vi "sample1.vi"() -> ()   [LabVIEW 2015]
uses:
  <vilib>/rvi/Emulation/niFpgaGetClockAttributes.vi
  <vilib>/rvi/Emulation/niFpgaSctlEmulationGetInTimedLoop.vi
  <vilib>/rvi/Emulation/niFpgaEmulationReportErrorSimple.vi
  <vilib>/rvi/eio/common/nirviEmuTemplateMethod_errors.vi
  <vilib>/rvi/Emulation/niFpgaCriticalErrorInLSC.vi
  <vilib>/rvi/Emulation/niFpgaProcessEmulError.vi
  <vilib>/eio/EIONode/EIONode.xnode
panel:
  in  "B Duty":u32 caption="Count(mSec)"
  in  "OR Duty":u32 caption="Count(mSec)"
  in  "OL Duty":u32 caption="Count(mSec)"
  in  "R duty":u32 caption="Count(mSec)"
  in  "Lights Period":u32
  in  "W duty":u32 caption="Count(mSec)"
  in  "Wiper Duty":u32 caption="Count(mSec)"
  in  "DoorB Duty":u32 caption="Count(mSec)"
  in  "Servo Period":u32
  in  "DoorA Duty":u32 caption="Count(mSec)"
  in  "Pulse Width":u32 caption="Count(mSec)"
  in  "Steering":i16
  in  "Stepper ON":bool
  in  "Period":u32=1
  in  "DIRECTION":bool
  in  "GAS":sgl
  in  "Count(mSec)":u32=1
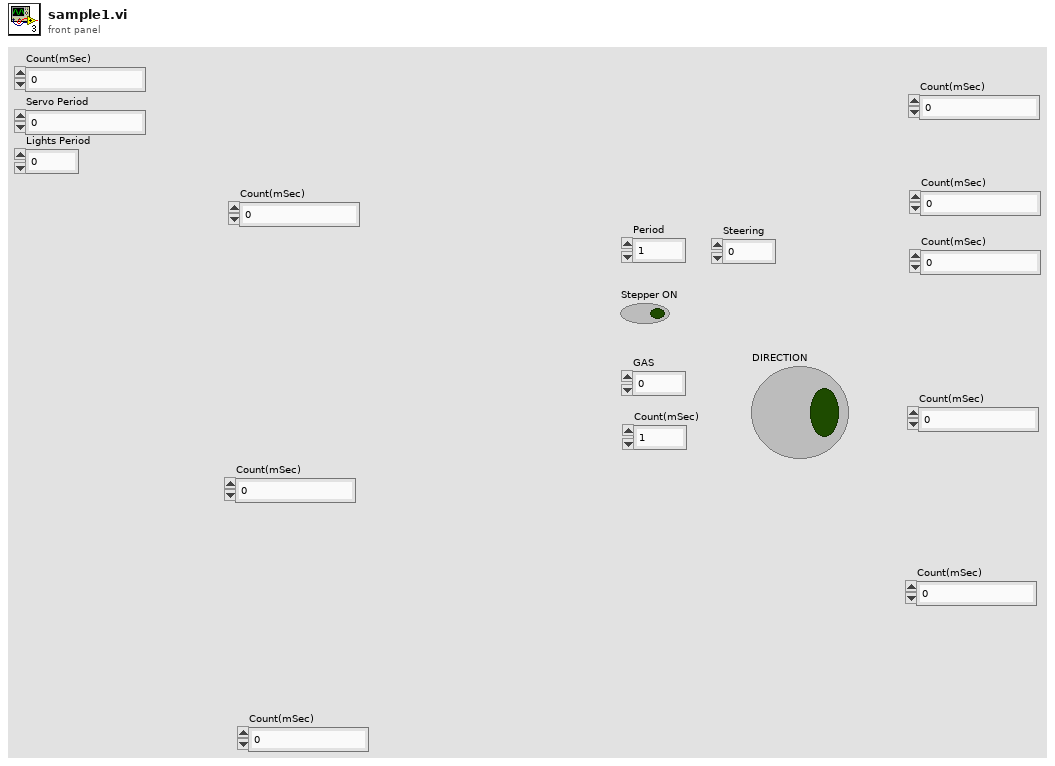
[diagram p1: front panel]
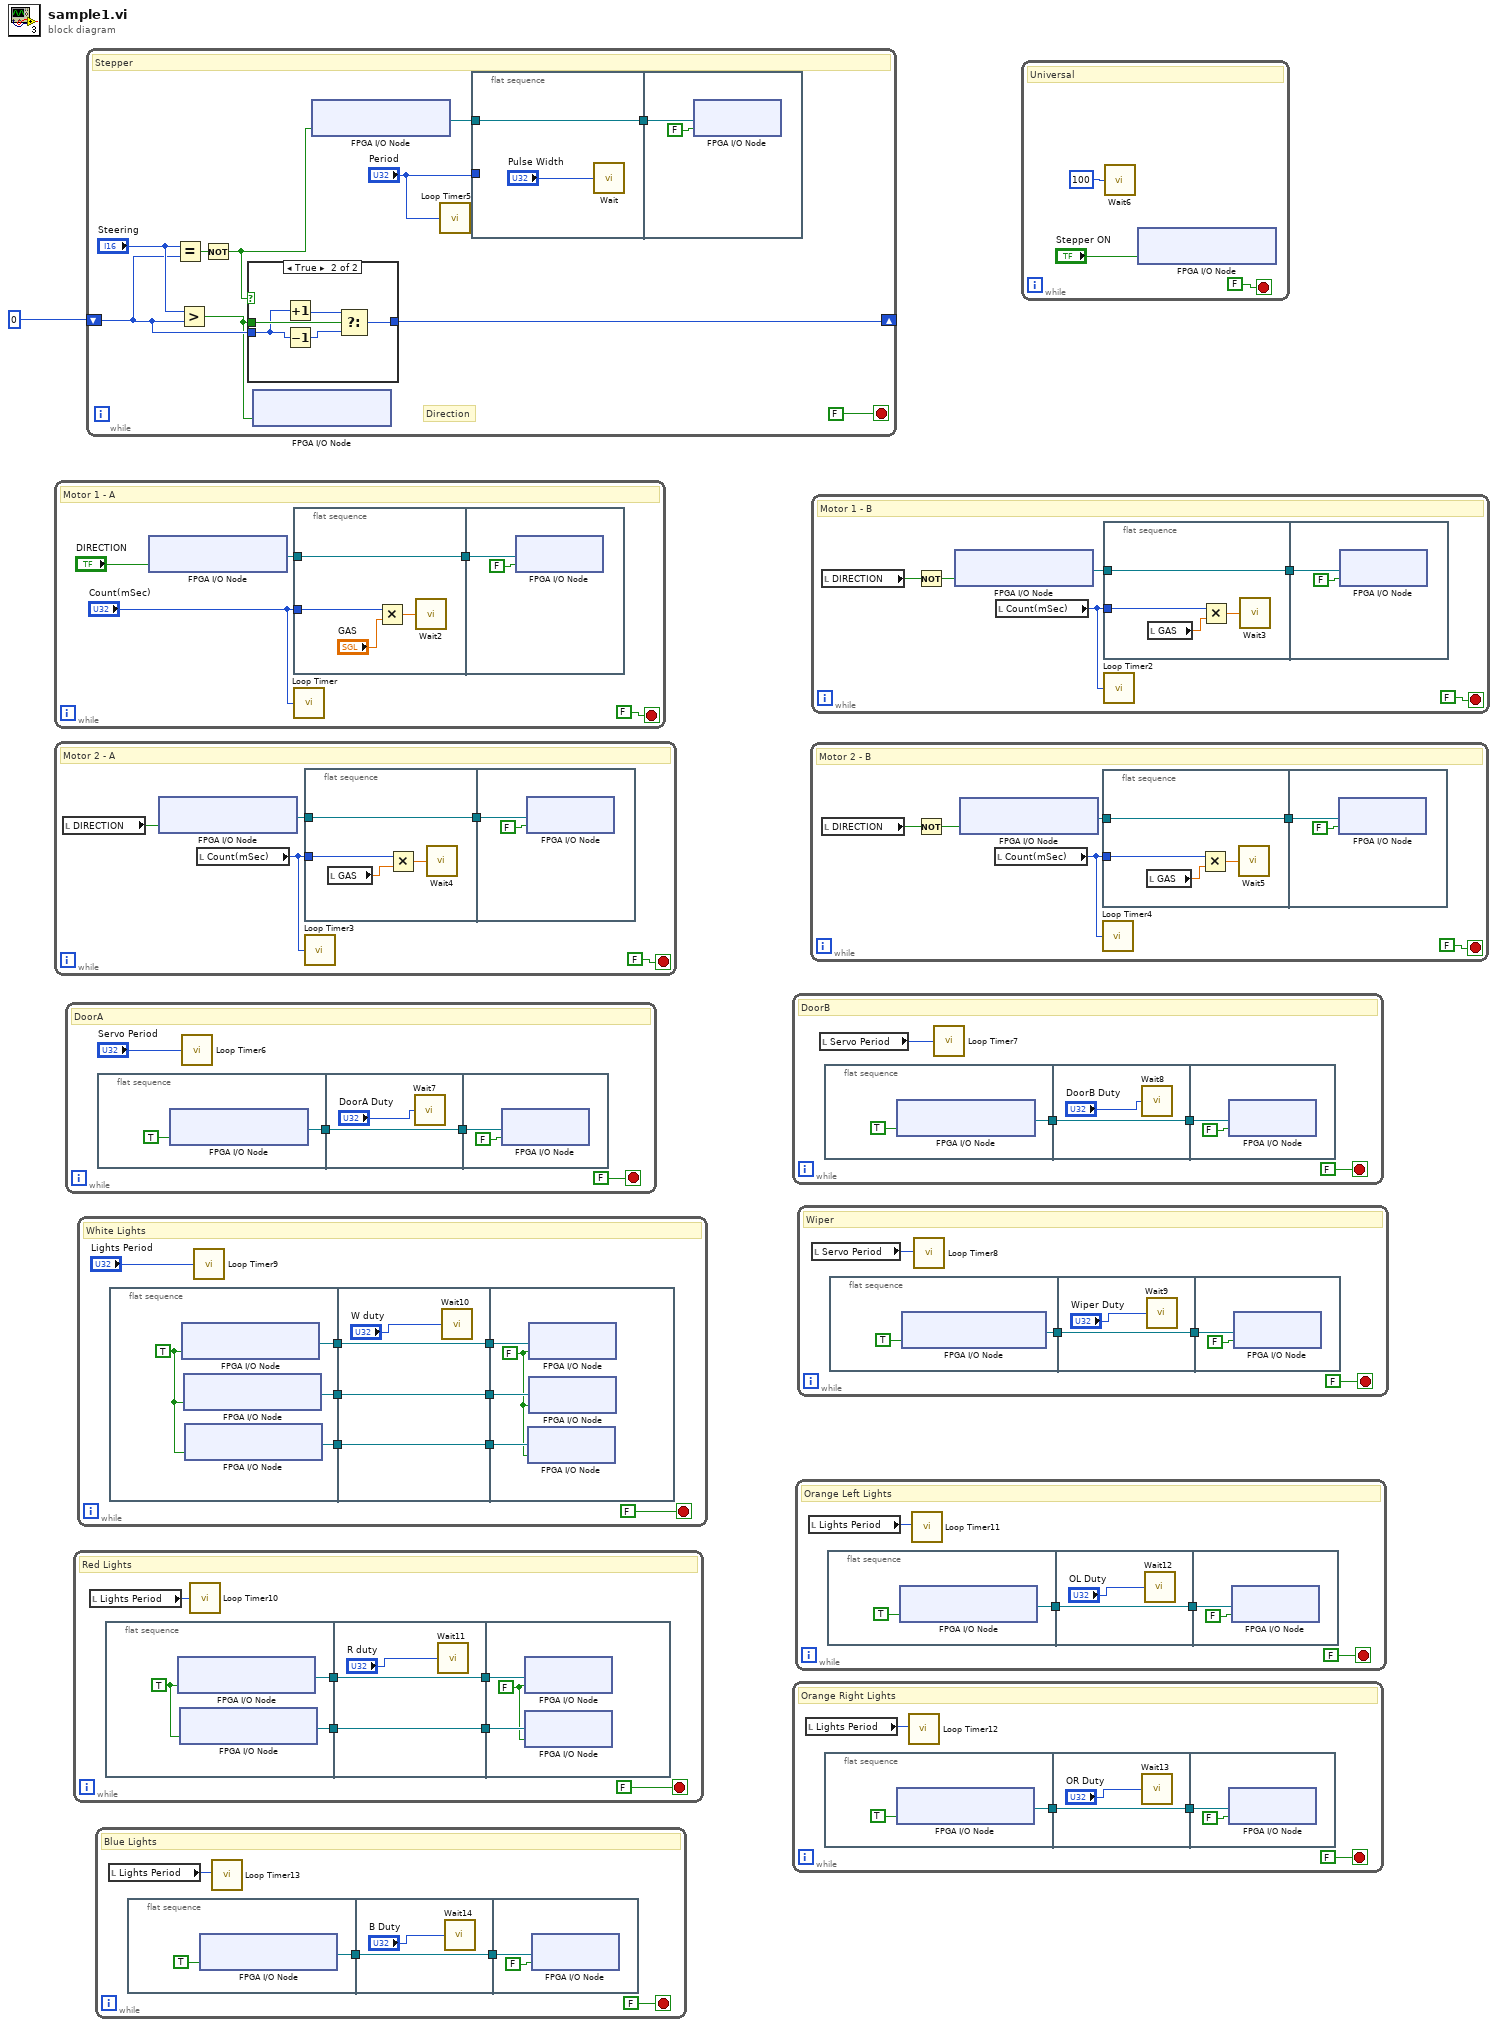
[diagram p0: block diagram]
diagram:
  n1 = while {
    stop <- FALSE stop-if-true
    # "Motor 1 - A"
    n2 = xnode "FPGA I/O Node"("ConnectorA/DIO0"="DIRECTION") -> ("FPGA I/O Out"=w5:refnum<k21>)  [unwired: 1 in]
    n3 = flat-sequence {
      tunnel: w5 -> [w8]
      tunnel: "Count(mSec)" -> [w10]
      tunnel: [w8] -> w3
      tunnel: w3 -> [w12]
      frame #0 {
        n4 = Multiply(x=w10, y="GAS") -> (x*y=w7:sgl)
        n5 = call "Wait2"("Count(mSec)"=w7) -> ()  [unwired: 1 out]
      }
      frame #1 {
        n6 = xnode "FPGA I/O Node"("I/O Item"=FALSE ("Mod5/DIO0"), "FPGA I/O In"=w12) -> ()  [unwired: 1 out]
      }
    }
    n7 = call "Loop Timer"("Count(mSec)"="Count(mSec)") -> ()  [unwired: 1 out]
  }
  n8 = while {
    stop <- FALSE stop-if-true
    # "Motor 2 - A"
    n9 = local read "DIRECTION"() -> (w14:bool)
    n10 = xnode "FPGA I/O Node"("ConnectorA/DIO2"=w14) -> ("FPGA I/O Out"=w16:refnum<k21>)  [unwired: 1 in]
    n11 = local read "Count(mSec)"() -> (w13:u32)
    n12 = flat-sequence {
      tunnel: w16 -> [w20]
      tunnel: w13 -> [w21]
      tunnel: [w20] -> w15
      tunnel: w15 -> [w23]
      frame #0 {
        n13 = local read "GAS"() -> (w18:sgl)
        n14 = Multiply(x=w21, y=w18) -> (x*y=w19:sgl)
        n15 = call "Wait4"("Count(mSec)"=w19) -> ()  [unwired: 1 out]
      }
      frame #1 {
        n16 = xnode "FPGA I/O Node"("I/O Item"=FALSE ("Mod5/DIO0"), "FPGA I/O In"=w23) -> ()  [unwired: 1 out]
      }
    }
    n17 = call "Loop Timer3"("Count(mSec)"=w13) -> ()  [unwired: 1 out]
  }
  n18 = while {
    stop <- FALSE stop-if-true
    # "DoorA"
    n19 = flat-sequence {
      tunnel: [w28] -> w25
      tunnel: [w30] -> w26
      tunnel: w25 -> [w30]
      tunnel: w26 -> [w32]
      frame #0 {
        n20 = xnode "FPGA I/O Node"("ConnectorA/DIO8"=TRUE) -> ("FPGA I/O Out"=w28:refnum<k21>)  [unwired: 1 in]
      }
      frame #1 {
        n21 = call "Wait7"("Count(mSec)"="DoorA Duty") -> ()  [unwired: 1 out]
      }
      frame #2 {
        n22 = xnode "FPGA I/O Node"("I/O Item"=FALSE ("ConnectorA/DIO8"), "FPGA I/O In"=w32) -> ()  [unwired: 1 out]
      }
    }
    n23 = call "Loop Timer6"("Count(mSec)"="Servo Period") -> ()  [unwired: 1 out]
  }
  n24 = while {
    stop <- FALSE stop-if-true
    # "Red Lights"
    n25 = local read "Lights Period"() -> (w34:u32)
    n26 = flat-sequence {
      tunnel: [w42] -> w38
      tunnel: [w40] -> w36
      tunnel: [w44] -> w39
      tunnel: w38 -> [w44]
      tunnel: w36 -> [w43]
      tunnel: [w43] -> w35
      tunnel: w39 -> [w48]
      tunnel: w35 -> [w47]
      frame #0 {
        w41 = TRUE ("ConnectorA/DIO8")
        n27 = xnode "FPGA I/O Node"("ConnectorB/DIO5"=w41) -> ("FPGA I/O Out"=w42:refnum<k21>)  [unwired: 1 in]
        n28 = xnode "FPGA I/O Node"("ConnectorB/DIO6"=w41) -> ("FPGA I/O Out"=w40:refnum<k21>)  [unwired: 1 in]
      }
      frame #1 {
        n29 = call "Wait11"("Count(mSec)"="R duty") -> ()  [unwired: 1 out]
      }
      frame #2 {
        w46 = FALSE ("ConnectorA/DIO8")
        n30 = xnode "FPGA I/O Node"("I/O Item"=w46, "FPGA I/O In"=w48) -> ()  [unwired: 1 out]
        n31 = xnode "FPGA I/O Node"("I/O Item"=w46, "FPGA I/O In"=w47) -> ()  [unwired: 1 out]
      }
    }
    n32 = call "Loop Timer10"("Count(mSec)"=w34) -> ()  [unwired: 1 out]
  }
  n33 = while {
    stop <- FALSE stop-if-true
    # "White Lights"
    n34 = flat-sequence {
      tunnel: [w60] -> w55
      tunnel: [w59] -> w52
      tunnel: [w58] -> w49
      tunnel: [w63] -> w56
      tunnel: w55 -> [w63]
      tunnel: w52 -> [w62]
      tunnel: [w62] -> w51
      tunnel: [w61] -> w50
      tunnel: w49 -> [w61]
      tunnel: w56 -> [w68]
      tunnel: w51 -> [w67]
      tunnel: w50 -> [w66]
      frame #0 {
        w57 = TRUE ("ConnectorA/DIO8")
        n35 = xnode "FPGA I/O Node"("ConnectorB/DIO0"=w57) -> ("FPGA I/O Out"=w60:refnum<k21>)  [unwired: 1 in]
        n36 = xnode "FPGA I/O Node"("ConnectorB/DIO1"=w57) -> ("FPGA I/O Out"=w59:refnum<k21>)  [unwired: 1 in]
        n37 = xnode "FPGA I/O Node"("ConnectorB/DIO2"=w57) -> ("FPGA I/O Out"=w58:refnum<k21>)  [unwired: 1 in]
      }
      frame #1 {
        n38 = call "Wait10"("Count(mSec)"="W duty") -> ()  [unwired: 1 out]
      }
      frame #2 {
        w65 = FALSE ("ConnectorA/DIO8")
        n39 = xnode "FPGA I/O Node"("I/O Item"=w65, "FPGA I/O In"=w66) -> ()  [unwired: 1 out]
        n40 = xnode "FPGA I/O Node"("I/O Item"=w65, "FPGA I/O In"=w68) -> ()  [unwired: 1 out]
        n41 = xnode "FPGA I/O Node"("I/O Item"=w65, "FPGA I/O In"=w67) -> ()  [unwired: 1 out]
      }
    }
    n42 = call "Loop Timer9"("Count(mSec)"="Lights Period") -> ()  [unwired: 1 out]
  }
  n43 = while {
    shift-right: [w69] -> _
    shift-left: i16 0 -> [w71]
    stop <- FALSE stop-if-true
    # "Direction"
    # "Stepper"
    n44 = Equal?(x="Steering", y=w71) -> (x = y?=w73:bool)
    n45 = Greater?(x="Steering", y=w71) -> (0:w70:bool)
    n46 = Not(x=w73) -> (.not. x?=w72:bool)
    n47 = case shown="True" w72 {
      tunnel: w71 -> [w79 w82]
      tunnel: w70 -> [_ w84]
      tunnel: [w79 w80] -> w69
      frame False {
      }
      frame True {
        n48 = Increment(x=w82) -> (x+1=w81:i16)
        n49 = Decrement(x=w82) -> (x-1=w83:i16)
        n50 = Select(t=w81, s=w84, f=w83) -> (s? t:f=w80:i16)
      }
    }
    n51 = xnode "FPGA I/O Node"("ConnectorA/DIO5"=w70) -> ()  [unwired: 1 in, 1 out]
    n52 = xnode "FPGA I/O Node"("ConnectorA/DIO4"=w72) -> ("FPGA I/O Out"=w76:refnum<k21>)  [unwired: 1 in]
    n53 = call "Loop Timer5"("Count(mSec)"="Period") -> ()  [unwired: 1 out]
    n54 = flat-sequence {
      tunnel: w76 -> [w86]
      tunnel: "Period" -> [_]
      tunnel: [w86] -> w77
      tunnel: w77 -> [w88]
      frame #0 {
        n55 = call "Wait"("Count(mSec)"="Pulse Width") -> ()  [unwired: 1 out]
      }
      frame #1 {
        n56 = xnode "FPGA I/O Node"("I/O Item"=FALSE ("Mod5/DIO0"), "FPGA I/O In"=w88) -> ()  [unwired: 1 out]
      }
    }
  }
  n57 = while {
    stop <- FALSE stop-if-true
    # "Blue Lights"
    n58 = local read "Lights Period"() -> (w89:u32)
    n59 = flat-sequence {
      tunnel: [w93] -> w91
      tunnel: [w95] -> w92
      tunnel: w91 -> [w95]
      tunnel: w92 -> [w97]
      frame #0 {
        n60 = xnode "FPGA I/O Node"("ConnectorB/DIO7"=TRUE ("ConnectorA/DIO8")) -> ("FPGA I/O Out"=w93:refnum<k21>)  [unwired: 1 in]
      }
      frame #1 {
        n61 = call "Wait14"("Count(mSec)"="B Duty") -> ()  [unwired: 1 out]
      }
      frame #2 {
        n62 = xnode "FPGA I/O Node"("I/O Item"=FALSE ("ConnectorA/DIO8"), "FPGA I/O In"=w97) -> ()  [unwired: 1 out]
      }
    }
    n63 = call "Loop Timer13"("Count(mSec)"=w89) -> ()  [unwired: 1 out]
  }
  n64 = while {
    stop <- FALSE stop-if-true
    # "DoorB"
    n65 = local read "Servo Period"() -> (w99:u32)
    n66 = flat-sequence {
      tunnel: [w103] -> w101
      tunnel: [w105] -> w102
      tunnel: w101 -> [w105]
      tunnel: w102 -> [w107]
      frame #0 {
        n67 = xnode "FPGA I/O Node"("ConnectorA/DIO9"=TRUE ("ConnectorA/DIO8")) -> ("FPGA I/O Out"=w103:refnum<k21>)  [unwired: 1 in]
      }
      frame #1 {
        n68 = call "Wait8"("Count(mSec)"="DoorB Duty") -> ()  [unwired: 1 out]
      }
      frame #2 {
        n69 = xnode "FPGA I/O Node"("I/O Item"=FALSE ("ConnectorA/DIO8"), "FPGA I/O In"=w107) -> ()  [unwired: 1 out]
      }
    }
    n70 = call "Loop Timer7"("Count(mSec)"=w99) -> ()  [unwired: 1 out]
  }
  n71 = while {
    stop <- FALSE stop-if-true
    # "Orange Right Lights"
    n72 = local read "Lights Period"() -> (w109:u32)
    n73 = flat-sequence {
      tunnel: [w113] -> w111
      tunnel: [w115] -> w112
      tunnel: w111 -> [w115]
      tunnel: w112 -> [w117]
      frame #0 {
        n74 = xnode "FPGA I/O Node"("ConnectorB/DIO4"=TRUE ("ConnectorA/DIO8")) -> ("FPGA I/O Out"=w113:refnum<k21>)  [unwired: 1 in]
      }
      frame #1 {
        n75 = call "Wait13"("Count(mSec)"="OR Duty") -> ()  [unwired: 1 out]
      }
      frame #2 {
        n76 = xnode "FPGA I/O Node"("I/O Item"=FALSE ("ConnectorA/DIO8"), "FPGA I/O In"=w117) -> ()  [unwired: 1 out]
      }
    }
    n77 = call "Loop Timer12"("Count(mSec)"=w109) -> ()  [unwired: 1 out]
  }
  n78 = while {
    stop <- FALSE stop-if-true
    # "Orange Left Lights"
    n79 = local read "Lights Period"() -> (w119:u32)
    n80 = flat-sequence {
      tunnel: [w123] -> w121
      tunnel: [w125] -> w122
      tunnel: w121 -> [w125]
      tunnel: w122 -> [w127]
      frame #0 {
        n81 = xnode "FPGA I/O Node"("ConnectorB/DIO3"=TRUE ("ConnectorA/DIO8")) -> ("FPGA I/O Out"=w123:refnum<k21>)  [unwired: 1 in]
      }
      frame #1 {
        n82 = call "Wait12"("Count(mSec)"="OL Duty") -> ()  [unwired: 1 out]
      }
      frame #2 {
        n83 = xnode "FPGA I/O Node"("I/O Item"=FALSE ("ConnectorA/DIO8"), "FPGA I/O In"=w127) -> ()  [unwired: 1 out]
      }
    }
    n84 = call "Loop Timer11"("Count(mSec)"=w119) -> ()  [unwired: 1 out]
  }
  n85 = while {
    stop <- FALSE stop-if-true
    # "Wiper"
    n86 = local read "Servo Period"() -> (w129:u32)
    n87 = flat-sequence {
      tunnel: [w133] -> w131
      tunnel: [w135] -> w132
      tunnel: w131 -> [w135]
      tunnel: w132 -> [w137]
      frame #0 {
        n88 = xnode "FPGA I/O Node"("ConnectorA/DIO10"=TRUE ("ConnectorA/DIO8")) -> ("FPGA I/O Out"=w133:refnum<k21>)  [unwired: 1 in]
      }
      frame #1 {
        n89 = call "Wait9"("Count(mSec)"="Wiper Duty") -> ()  [unwired: 1 out]
      }
      frame #2 {
        n90 = xnode "FPGA I/O Node"("I/O Item"=FALSE ("ConnectorA/DIO8"), "FPGA I/O In"=w137) -> ()  [unwired: 1 out]
      }
    }
    n91 = call "Loop Timer8"("Count(mSec)"=w129) -> ()  [unwired: 1 out]
  }
  n92 = while {
    stop <- FALSE stop-if-true
    # "Motor 2 - B"
    n93 = local read "DIRECTION"() -> (w141:bool)
    n94 = Not(x=w141) -> (.not. x?=w140:bool)
    n95 = xnode "FPGA I/O Node"("ConnectorA/DIO3"=w140) -> ("FPGA I/O Out"=w143:refnum<k21>)  [unwired: 1 in]
    n96 = local read "Count(mSec)"() -> (w139:u32)
    n97 = flat-sequence {
      tunnel: w143 -> [w147]
      tunnel: w139 -> [w148]
      tunnel: [w147] -> w142
      tunnel: w142 -> [w150]
      frame #0 {
        n98 = local read "GAS"() -> (w145:sgl)
        n99 = Multiply(x=w148, y=w145) -> (x*y=w146:sgl)
        n100 = call "Wait5"("Count(mSec)"=w146) -> ()  [unwired: 1 out]
      }
      frame #1 {
        n101 = xnode "FPGA I/O Node"("I/O Item"=FALSE ("Mod5/DIO0"), "FPGA I/O In"=w150) -> ()  [unwired: 1 out]
      }
    }
    n102 = call "Loop Timer4"("Count(mSec)"=w139) -> ()  [unwired: 1 out]
  }
  n103 = while {
    stop <- FALSE stop-if-true
    # "Motor 1 - B"
    n104 = local read "DIRECTION"() -> (w153:bool)
    n105 = Not(x=w153) -> (.not. x?=w152:bool)
    n106 = xnode "FPGA I/O Node"("ConnectorA/DIO1"=w152) -> ("FPGA I/O Out"=w155:refnum<k21>)  [unwired: 1 in]
    n107 = local read "Count(mSec)"() -> (w151:u32)
    n108 = flat-sequence {
      tunnel: w155 -> [w159]
      tunnel: w151 -> [w160]
      tunnel: [w159] -> w154
      tunnel: w154 -> [w162]
      frame #0 {
        n109 = local read "GAS"() -> (w157:sgl)
        n110 = Multiply(x=w160, y=w157) -> (x*y=w158:sgl)
        n111 = call "Wait3"("Count(mSec)"=w158) -> ()  [unwired: 1 out]
      }
      frame #1 {
        n112 = xnode "FPGA I/O Node"("I/O Item"=FALSE ("Mod5/DIO0"), "FPGA I/O In"=w162) -> ()  [unwired: 1 out]
      }
    }
    n113 = call "Loop Timer2"("Count(mSec)"=w151) -> ()  [unwired: 1 out]
  }
  n114 = while {
    stop <- FALSE stop-if-true
    # "Universal"
    n115 = call "Wait6"("Count(mSec)"=u32 100) -> ()  [unwired: 1 out]
    n116 = xnode "FPGA I/O Node"("ConnectorA/DIO6"="Stepper ON") -> ()  [unwired: 1 in, 1 out]
  }
